vi "PID Autotuning Design (Ziegler-Nichols).vi"(5 "Ziegler-Nichols Speed":u16(ring) items=["Fast", "Normal", "Slow"], 6 "Controller Gain (K)":dbl, 7 "Type of Controller":u16(ring) items=["P", "PI", "PID"], 8 "dt (s)":dbl, 9 "closed-loop?":bool, 10 "Response signal":dbl[](array[numeric]), 11 "Stimulus signal":dbl[](array[numeric])) -> (1 "PID gains":T2, 2 "response operating point":dbl, 3 "stimulus operating point":dbl, 4 "Plant Parameters":T1)   [LabVIEW 2020, in "NI_PID_autopid.lvlib"]
doc: "Implements autotuning using the tuning method associated with the polymorphic instance you select. This VI generates PID parameters based on the <B>Stimulus signal</B> and <B>Response signal</B> you specify. You can use this VI to generate initial parameters when you do not have sufficient information about the system you want to tune. You must manually select the polymorphic instance to use."
uses:
  <vilib>/addons/control/pid/NI_PID_autopid.lvlib
  <vilib>/addons/control/pid/NI_PID_pid.lvlib
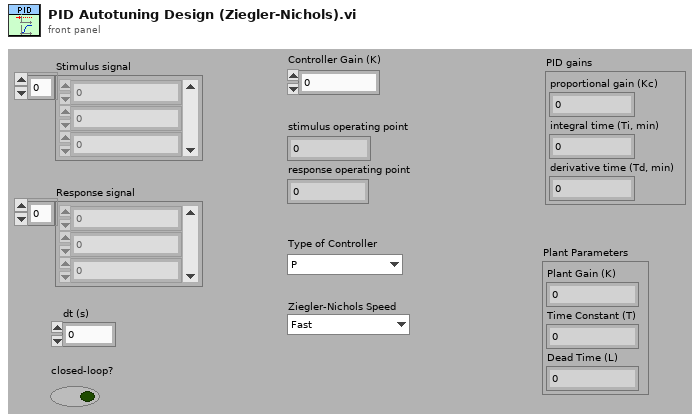
[diagram p1: front panel]
types:
  T1 = cluster{"Plant Gain (K)":dbl, "Time Constant (T)":dbl, "Dead Time (L)":dbl}
  T2 = cluster{"proportional gain (Kc)":dbl, "integral time (Ti, min)":dbl, "derivative time (Td, min)":dbl}
  T3 = enum16{"Academic (Standard)", "Parallel", "Series"}
  T4 = cluster{"OL Gain (Kp)":dbl, "OL Time Constant (T)":dbl, "Dead Time (L) Out":dbl}
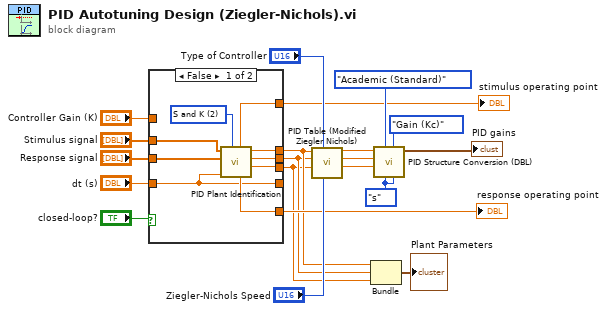
[diagram p0: block diagram]
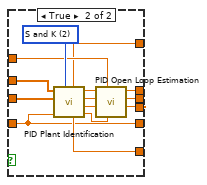
[diagram p2: hidden frame]
diagram:
  w13 = enum16{"min", "s"}."s" ("Integral Unit")
  n1 = case shown="False" "closed-loop?" {
    tunnel: "Response signal" -> [w28 w41]
    tunnel: "Stimulus signal" -> [w27 w42]
    tunnel: [w26 w33] -> w9
    tunnel: [w25 w32] -> w8
    tunnel: [w24 w39] -> w7
    tunnel: [w23 w40] -> w6
    tunnel: [w22 w31] -> w5
    tunnel: "dt (s)" -> [w21 w30]
    tunnel: "Controller Gain (K)" -> [_ w34]
    tunnel: [w21 w30] -> _
    frame False {
      w29 = u16 2 items=["Z-N", "First Order", "S and K"] ("Ring")
      n2 = call <vilib>:"PID Plant Identification.vi"("Method"=w29, "Sampling Time"=w21, "Response signal"=w28, "Stimulus signal"=w27) -> ("Dead Time (L)"=w22:dbl, "Time Constant (T)"=w23:dbl, "Plant Gain (K)"=w24:dbl, "response offset"=w25:dbl, "stimulus offset"=w26:dbl)  [unwired: 1 in, 2 out]
    }
    frame True {
      w43 = u16 2 items=["Z-N", "First Order", "S and K", "Second Order"] ("Method")
      n3 = call <vilib>:"PID Plant Identification.vi"("Method"=w43, "Sampling Time"=w30, "Response signal"=w41, "Stimulus signal"=w42) -> ("Time Constant (T) 2"=w35:dbl, "Dead Time (L)"=w36:dbl, "Time Constant (T)"=w37:dbl, "Plant Gain (K)"=w38:dbl, "response offset"=w32:dbl, "stimulus offset"=w33:dbl)  [unwired: 1 in, 1 out]
      n4 = call <vilib>:"PID Open Loop Estimation.vi"("CL Time Constant (T) 2"=w35, "Controller Gain (K)"=w34, "Dead Time (L)"=w36, "CL Time Constant (Tcl)"=w37, "CL Gain (Kcl)"=w38) -> ("Dead Time (L) Out"=w31:dbl, "OL Time Constant (T)"=w40:dbl, "OL Gain (Kp)"=w39:dbl)  [unwired: 4 in]
    }
  }
  "stimulus operating point" <- w9
  "response operating point" <- w8
  n5 = call <vilib>:"PID Table (Modified Ziegler Nichols).vi"("Ziegler-Nichlos Speed"="Ziegler-Nichols Speed", "Type of Controller"="Type of Controller", "Dead Time (L)"=w5, "Time Constant (T)"=w6, "Plant Gain (K)"=w7) -> ("Derivative Time (Td)"=w16:dbl, "Integral Time (Ti)"=w17:dbl, "Proportional Gain (Kp)"=w18:dbl)  [unwired: 4 in]
  n6 = Bundle("OL Gain (Kp)"=w7, "OL Time Constant (T)"=w6, "Dead Time (L) Out"=w5) -> (→"Plant Parameters":T4)  [unwired: 1 in]
  n7 = call <vilib>:"PID Structure Conversion (DBL).vi"("derivative unit"=w13, "proportional unit"=enum16{"Gain (Kc)", "Band (PB)"}."Gain (Kc)" ("Proportional Unit"), "integral unit"=w13, "PID structure"=T3."Academic (Standard)" ("PID Structure"), "derivative"=w16, "integral"=w17, "proportional"=w18) -> ("PID gains"=→"PID gains":T2)  [unwired: 4 in]
